vi "Clear myTemp.vi"(8 "error in (no error)":errorcluster, 11 "task array in":refnum<k21>[](array[refnum])) -> (0 "error out":errorcluster)   [LabVIEW 2013]
doc: "Turns the myTemp Digital lines off and clears both myTemp tasks."
uses:
  <vilib>/DAQmx/write.llb/DAQmx Write (Digital 1D Bool NChan 1Samp 1Line).vi
  <vilib>/DAQmx/miscellaneous.llb/DAQmx Fill In Error Info.vi
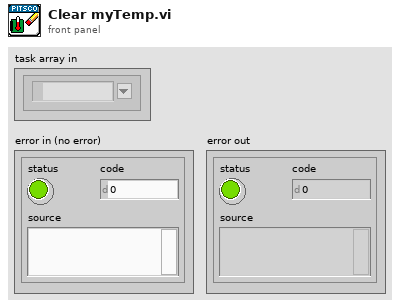
[diagram p1: front panel]
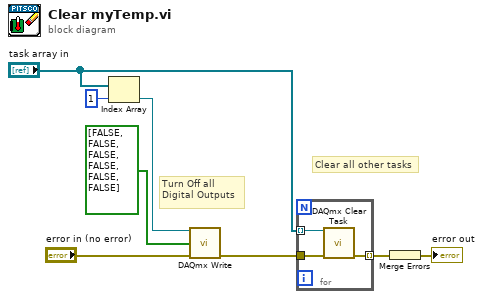
[diagram p0: block diagram]
diagram:
  # "Clear all other tasks"
  # "Turn Off all Digital Outputs"
  n1 = Index Array(array="task array in", index=1) -> (element=w6:refnum<k21>)
  n2 = call-poly <vilib>:"DAQmx Write.vi"("task/channels in"=w6, "data"=bool[] [FALSE, FALSE, FALSE, FALSE, FALSE, FALSE], "error in"="error in (no error)") -> ("error out"=w7:errorcluster)  [unwired: 10 in, 2 out]
  n3 = for {
    tunnel: w7 -> [w11]
    tunnel: "task array in" -> [w10] mode=indexing
    tunnel: [w9] -> w8 mode=indexing
    n4 = call <vilib>:"DAQmx Clear Task.vi"("task in"=w10, "error in"=w11) -> ("error out"=w9:errorcluster)  [unwired: 13 in]
  }
  n5 = Merge Errors(w8) -> (→"error out":errorcluster)
